vi "List alarmList.vi"(8 "error in (no error)":errorcluster) -> (0 "error out":errorcluster, 2 "columns":string[](array[string]), 3 "data":string[][](array[string]))   [LabVIEW 2016, in "Alarm interface.lvlib"]
uses:
  Alarm interface.lvlib
  <vilib>/addons/database/_DB Variant To Data/Database Variant To Data.xnode
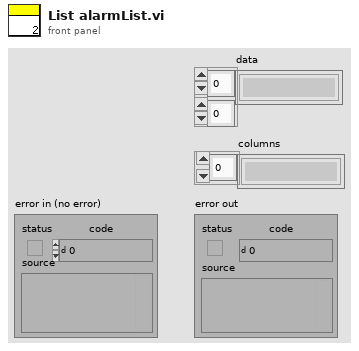
[diagram p1: front panel]
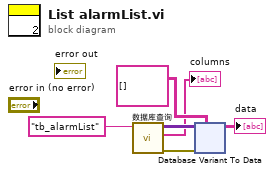
[diagram p0: block diagram]
diagram:
  n1 = call "数据库查询.vi"("table"="tb_alarmList") -> ("error out"=w3:errorcluster, "columns 2"=→"columns":string[], "data"=w5:variant[][])  [unwired: 8 in]
  n2 = xnode "Database Variant To Data"("database variant"=w5, "error in (no error)"=w3, "type"=string[][] []) -> ("data"=→"data":string[][])  [unwired: 1 out]
